vi "gentec-SOLO-PE.Query Configuration.vi"(8 "error in (no error)":errorcluster, 11 "VISA Refnum in":refnum<visa-resource-name>) -> (0 "error out":errorcluster, 1 "Configuration":T1 {"Reference Value" format="%.6f"; "Lower Bond" format="%.6f"; "Upper Bound" format="%.6f"; "Resolution" format="%.7f"; "Max energy (Joulemeter)" format="%.6f"; "Max Power (Joulemeter)" format="%.6f"; "Offset 2" format="%.6f"; "Multiplier 2" format="%.6f"; "Offset 1" format="%.6f"; "Multiplier 1" format="%.6f"; "Zero Offset" format="%.6f"; "Trig Level" format="%.6f"; "Current Scale" items=["Auto", "1 pJ", "3 pJ", "10 pJ", "30 pJ", "100 pJ", "300 pJ", "1 nJ", "3 nJ", "10 nJ", "30 nJ", "100 nJ", "300 nJ", "1 uJ", "3 uJ", "10 uJ", "30 uJ", "100 uJ", "300 uJ", "1 mJ", "3 mJ", "10 mJ", "30 mJ", "100 mJ", "300 mJ", "1 J", "3 J", "10 J", "30 J", "100 J", "300 J", "1 kJ", "3 kJ", "10 kJ", "30 kJ", "100 kJ", "300 kJ", "1 MJ", "3 MJ", "10 MJ", "30 MJ", "100 MJ", "300 MJ"]; "Scale Max Energy" items=["Auto", "1 pJ", "3 pJ", "10 pJ", "30 pJ", "100 pJ", "300 pJ", "1 nJ", "3 nJ", "10 nJ", "30 nJ", "100 nJ", "300 nJ", "1 uJ", "3 uJ", "10 uJ", "30 uJ", "100 uJ", "300 uJ", "1 mJ", "3 mJ", "10 mJ", "30 mJ", "100 mJ", "300 mJ", "1 J", "3 J", "10 J", "30 J", "100 J", "300 J", "1 kJ", "3 kJ", "10 kJ", "30 kJ", "100 kJ", "300 kJ", "1 MJ", "3 MJ", "10 MJ", "30 MJ", "100 MJ", "300 MJ"]; "Scale Min Energy" items=["Auto", "1 pJ", "3 pJ", "10 pJ", "30 pJ", "100 pJ", "300 pJ", "1 nJ", "3 nJ", "10 nJ", "30 nJ", "100 nJ", "300 nJ", "1 uJ", "3 uJ", "10 uJ", "30 uJ", "100 uJ", "300 uJ", "1 mJ", "3 mJ", "10 mJ", "30 mJ", "100 mJ", "300 mJ", "1 J", "3 J", "10 J", "30 J", "100 J", "300 J", "1 kJ", "3 kJ", "10 kJ", "30 kJ", "100 kJ", "300 kJ", "1 MJ", "3 MJ", "10 MJ", "30 MJ", "100 MJ", "300 MJ"]; "Active Sensitivity" format="%.6f"; "Calibration Sensitivity" format="%.6f"}, 2 "Error":string, 3 "VISA Refnum out":refnum<visa-resource-name>, 4 "Timeout":bool)   [LabVIEW 2014, in "gentec-SOLO-PE - Driver.lvlib"]
doc: "Queries the Configuration."
uses:
  gentec-SOLO-PE - Driver.lvlib
  Type Defs/gentec-SOLO-PE.Configuration Values.ctl
  Type Defs/gentec-SOLO-PE.Scale.ctl
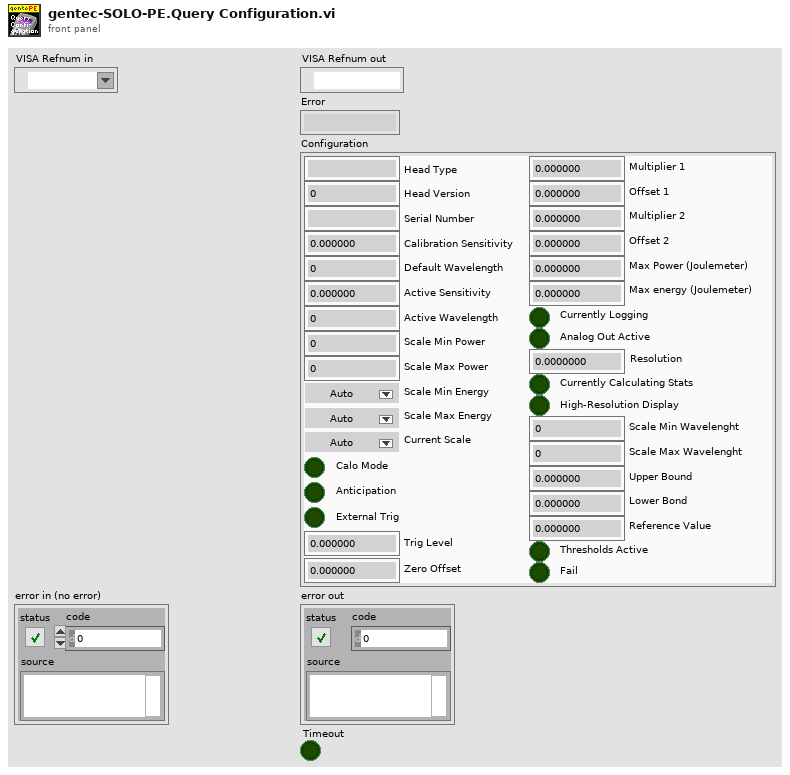
[diagram p1: front panel]
types:
  T1 = typedef "gentec-SOLO-PE - Driver.lvlib/gentec-SOLO-PE.Configuration Values.ctl" = cluster{"Head Type":string, "Head Version":u32, "Serial Number":string, "Calibration Sensitivity":dbl, "Default Wavelength":u32, "Active Sensitivity":dbl, "Active Wavelength":u32, "Scale Min Power":u32, "Scale Max Power":u32, "Scale Min Energy":T2, "Scale Max Energy":T2, "Current Scale":T2, "Calo Mode":bool, "Anticipation":bool, "External Trig":bool, "Trig Level":dbl, "Zero Offset":dbl, "Multiplier 1":dbl, "Offset 1":dbl, "Multiplier 2":dbl, "Offset 2":dbl, "Max Power (Joulemeter)":dbl, "Max energy (Joulemeter)":dbl, "Currently Logging":bool, "Analog Out Active":bool, "Resolution":dbl, "Currently Calculating Stats":bool, "High-Resolution Display":bool, "Scale Min Wavelenght":u32, "Scale Max Wavelenght":u32, "Upper Bound":dbl, "Lower Bond":dbl, "Reference Value":dbl, "Thresholds Active":bool, "Fail":bool}
  T2 = typedef "gentec-SOLO-PE - Driver.lvlib/gentec-SOLO-PE.Scale.ctl" = u32
  T3 = cluster{"Return Parameters[0]":u32, "Return Parameters[1]":u32, "Return Parameters[2]":u32, "Return Parameters[3]":u32, "Return Parameters[4]":u32, "Return Parameters[5]":u32, "Return Parameters[6]":u32, "Return Parameters[7]":u32, "Return Parameters[8]":u32, "Return Parameters[9]":u32, "Return Parameters[10]":u32, "Return Parameters[11]":u32, "Return Parameters[12]":u32, "Return Parameters[13]":u32, "Return Parameters[14]":u32, "Return Parameters[15]":u32, "Return Parameters[16]":u32, "Return Parameters[17]":u32, "Return Parameters[18]":u32, "Return Parameters[19]":u32, "Return Parameters[20]":u32, "Return Parameters[21]":u32, "Return Parameters[22]":u32, "Return Parameters[23]":u32, "Return Parameters[24]":u32, "Return Parameters[25]":u32, "Return Parameters[26]":u32, "Return Parameters[27]":u32, "Return Parameters[28]":u32, "Return Parameters[29]":u32, "Return Parameters[30]":u32, "Return Parameters[31]":u32, "Return Parameters[32]":u32, "Return Parameters[33]":u32, "Return Parameters[34]":u32, "Return Parameters[35]":u32, "Return Parameters[36]":u32, "Return Parameters[37]":u32, "Return Parameters[38]":u32, "Return Parameters[39]":u32, "Return Parameters[40]":u32, "Return Parameters[41]":u32}
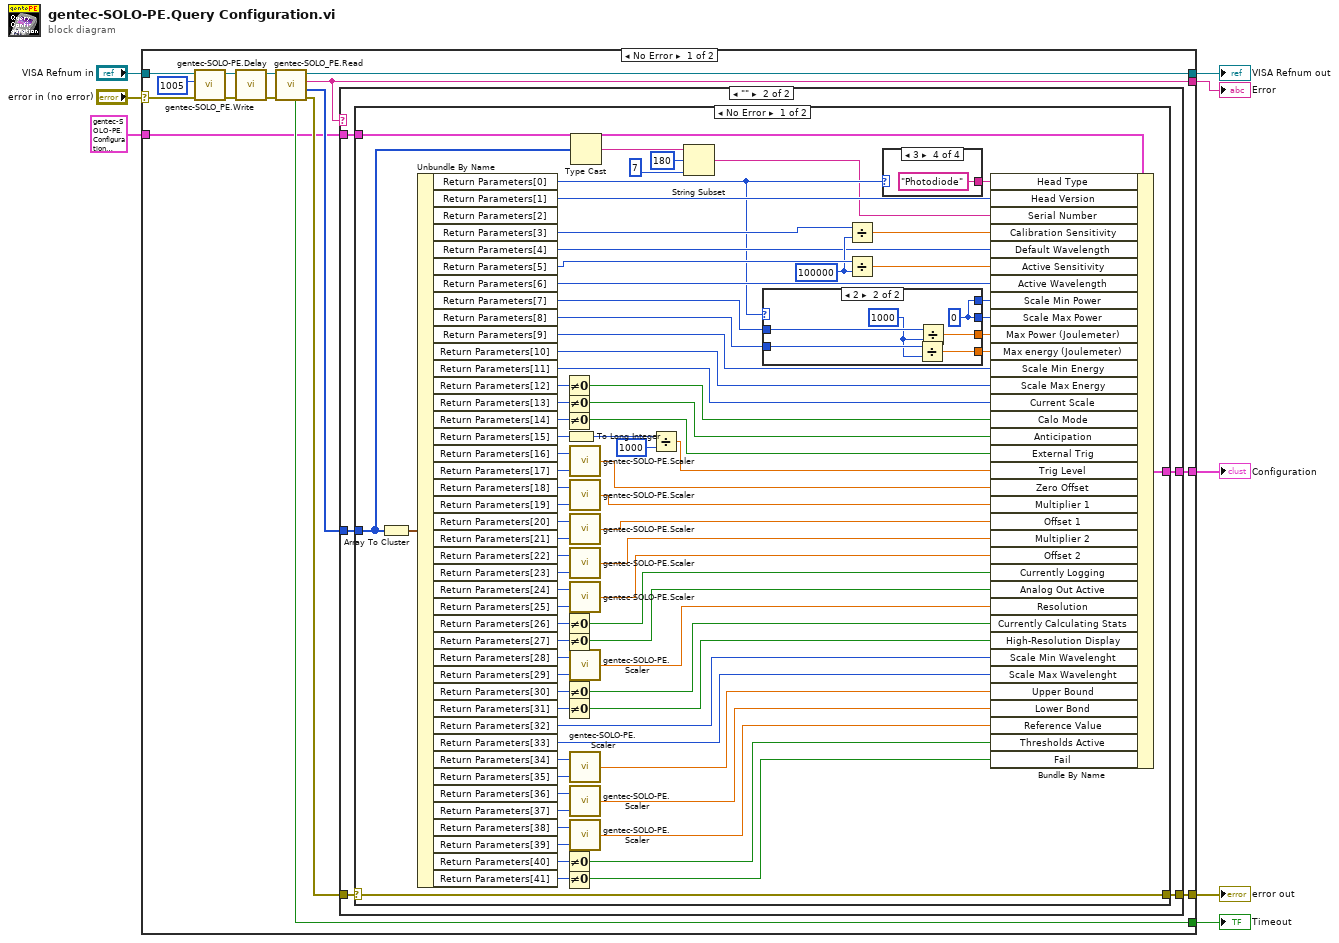
[diagram p0: block diagram]
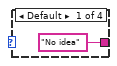
[diagram p3: hidden frame]
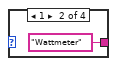
[diagram p4: hidden frame]
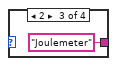
[diagram p5: hidden frame]
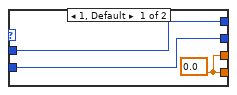
[diagram p6: hidden frame]
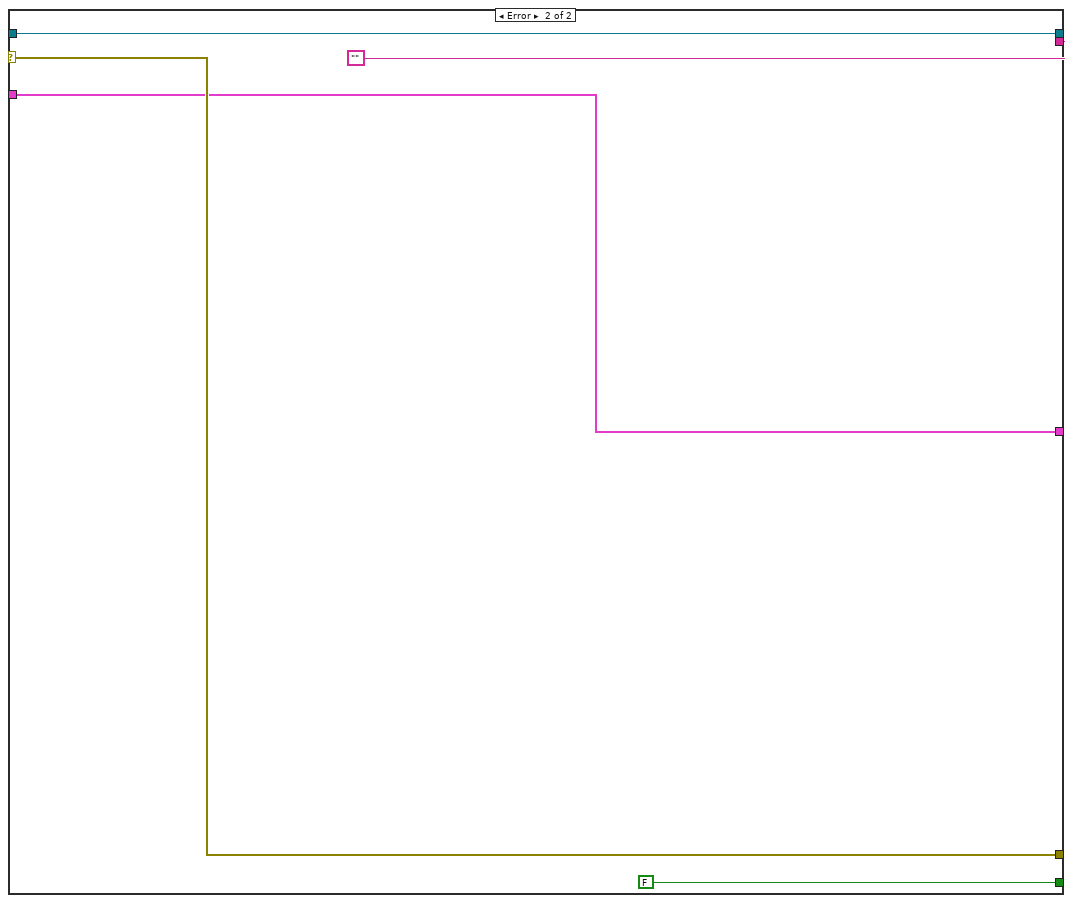
[diagram p8: hidden frame]
diagram:
  n1 = case shown="No Error" "error in (no error)" {
    selector: "error in (no error)" -> [w15 w128]
    tunnel: [w12 w128] -> w8
    tunnel: [w23 w129] -> w7
    tunnel: [w11 ""] -> w6
    tunnel: [w22 FALSE ("Timeout")] -> w5
    tunnel: "VISA Refnum in" -> [w17 w129]
    tunnel: [w10 w125] -> w2
    tunnel: T1 {"Head Type"="", "Head Version"=0, "Serial Number"="", "Calibration Sensitivity"=0.0, "Default Wavelength"=0, "Active Sensitivity"=0.0, "Active Wavelength"=0, "Scale Min Power"=0, "Scale Max Power"=0, "Scale Min Energy"=0, "Scale Max Energy"=0, "Current Scale"=0, "Calo Mode"=FALSE, "Anticipation"=FALSE, "External Trig"=FALSE, "Trig Level"=0.0, "Zero Offset"=0.0, "Multiplier 1"=0.0, "Offset 1"=0.0, "Multiplier 2"=0.0, "Offset 2"=0.0, "Max Power (Joulemeter)"=0.0, "Max energy (Joulemeter)"=0.0, "Currently Logging"=FALSE, "Analog Out Active"=FALSE, "Resolution"=0.0, "Currently Calculating Stats"=FALSE, "High-Resolution Display"=FALSE, "Scale Min Wavelenght"=0, "Scale Max Wavelenght"=0, "Upper Bound"=0.0, "Lower Bond"=0.0, "Reference Value"=0.0, "Thresholds Active"=FALSE, "Fail"=FALSE} ("Configuration") -> [w9 w125]
    frame No Error {
      n2 = call "gentec-SOLO_PE.Write.vi"("error in (no error)"=w15, "Command Handle"=u16 1005, "VISA Refnum in"=w17) -> ("error out"=w20:errorcluster, "VISA Refnum out"=w18:refnum<visa-resource-name>)  [unwired: 7 in]
      n3 = call "gentec-SOLO-PE.Delay.vi"("error in (no error)"=w20, "VISA resource In"=w18) -> ("error out"=w21:errorcluster, "VISA resource Out"=w19:refnum<visa-resource-name>)  [unwired: 4 in]
      n4 = call "gentec-SOLO_PE.Read.vi"("error in (no error)"=w21, "VISA Refnum in"=w19) -> ("error out"=w13:errorcluster, "Return Parameters"=w14:u32[], "Error"=w11:string, "VISA Refnum out"=w23:refnum<visa-resource-name>, "Timeout"=w22:bool)  [unwired: 5 in]
      n5 = case shown="\"\"" w11 {
        tunnel: w14 -> [_ w30]
        tunnel: w13 -> [w25 w29]
        tunnel: [w25 w28] -> w12
        tunnel: w9 -> [w24 w27]
        tunnel: [w24 w26] -> w10
        frame Default {
        }
        frame "" {
          n6 = case shown="No Error" w29 {
            selector: w29 -> [w109 w124]
            tunnel: w30 -> [w34 _]
            tunnel: [w109 w124] -> w28
            tunnel: w27 -> [w44 w123]
            tunnel: [w41 w123] -> w26
            frame No Error {
              w100 = 100000
              n7 = Array To Cluster(array=w34) -> (cluster=w47:T3)
              n8 = Unbundle By Name(w47) -> ("Return Parameters[0]"=w43:u32, "Return Parameters[1]"=w75:u32, "Return Parameters[3]"=w101:u32, "Return Parameters[4]"=w73:u32, "Return Parameters[5]"=w108:u32, "Return Parameters[6]"=w71:u32, "Return Parameters[7]"=w104:u32, "Return Parameters[8]"=w103:u32, "Return Parameters[9]"=w38:u32, "Return Parameters[10]"=w70:u32, "Return Parameters[11]"=w69:u32, "Return Parameters[12]"=w107:u32, "Return Parameters[13]"=w106:u32, "Return Parameters[14]"=w105:u32, "Return Parameters[15]"=w97:u32, "Return Parameters[16]"=w90:u32, "Return Parameters[17]"=w91:u32, "Return Parameters[18]"=w89:u32, "Return Parameters[19]"=w46:u32, "Return Parameters[20]"=w45:u32, "Return Parameters[21]"=w88:u32, "Return Parameters[22]"=w86:u32, "Return Parameters[23]"=w87:u32, "Return Parameters[24]"=w84:u32, "Return Parameters[25]"=w85:u32, "Return Parameters[26]"=w102:u32, "Return Parameters[27]"=w99:u32, "Return Parameters[28]"=w83:u32, "Return Parameters[29]"=w82:u32, "Return Parameters[30]"=w95:u32, "Return Parameters[31]"=w94:u32, "Return Parameters[32]"=w54:u32, "Return Parameters[33]"=w53:u32, "Return Parameters[34]"=w81:u32, "Return Parameters[35]"=w80:u32, "Return Parameters[36]"=w79:u32, "Return Parameters[37]"=w78:u32, "Return Parameters[38]"=w77:u32, "Return Parameters[39]"=w76:u32, "Return Parameters[40]"=w93:u32, "Return Parameters[41]"=w92:u32)  [unwired: 1 out]
              n9 = Not Equal To 0?(x=w107) -> (x != 0?=w68:bool)
              n10 = Not Equal To 0?(x=w106) -> (x != 0?=w67:bool)
              n11 = Not Equal To 0?(x=w105) -> (x != 0?=w66:bool)
              n12 = Not Equal To 0?(x=w102) -> (x != 0?=w59:bool)
              n13 = Not Equal To 0?(x=w99) -> (x != 0?=w58:bool)
              n14 = Not Equal To 0?(x=w95) -> (x != 0?=w56:bool)
              n15 = Not Equal To 0?(x=w94) -> (x != 0?=w55:bool)
              n16 = Not Equal To 0?(x=w93) -> (x != 0?=w49:bool)
              n17 = Not Equal To 0?(x=w92) -> (x != 0?=w48:bool)
              n18 = To Long Integer(number=w97) -> (32bit integer=w98:i32)
              n19 = call "gentec-SOLO-PE.Scaler.vi"("Scaler"=w91, "Value"=w90) -> ("Scaled Value"=w64:dbl)
              n20 = call "gentec-SOLO-PE.Scaler.vi"("Scaler"=w46, "Value"=w89) -> ("Scaled Value"=w63:dbl)
              n21 = call "gentec-SOLO-PE.Scaler.vi"("Scaler"=w88, "Value"=w45) -> ("Scaled Value"=w62:dbl)
              n22 = call "gentec-SOLO-PE.Scaler.vi"("Scaler"=w87, "Value"=w86) -> ("Scaled Value"=w61:dbl)
              n23 = call "gentec-SOLO-PE.Scaler.vi"("Scaler"=w85, "Value"=w84) -> ("Scaled Value"=w60:dbl)
              n24 = call "gentec-SOLO-PE.Scaler.vi"("Scaler"=w82, "Value"=w83) -> ("Scaled Value"=w57:dbl)
              n25 = call "gentec-SOLO-PE.Scaler.vi"("Scaler"=w80, "Value"=w81) -> ("Scaled Value"=w52:dbl)
              n26 = call "gentec-SOLO-PE.Scaler.vi"("Scaler"=w78, "Value"=w79) -> ("Scaled Value"=w51:dbl)
              n27 = call "gentec-SOLO-PE.Scaler.vi"("Scaler"=w76, "Value"=w77) -> ("Scaled Value"=w50:dbl)
              n28 = Type Cast(x=w34) -> (*(type *) &x=w33:string)  [unwired: 1 in]
              n29 = Divide(x=w98, y=1000) -> (x/y=w65:dbl)
              n30 = String Subset(string=w33, offset (0)=180, length (rest)=7 ("length (rest)")) -> (substring=w31:string)
              n31 = case shown="2" w43 {
                tunnel: w104 -> [w116 w121]
                tunnel: w103 -> [w115 w120]
                tunnel: [w116 w122] -> w40
                tunnel: [w115 w122] -> w39
                tunnel: [w114 w119] -> w37
                tunnel: [w114 w118] -> w36
                frame 1, Default {
                  w114 = 0.0
                }
                frame 2 {
                  w117 = 1000
                  w122 = 0
                  n32 = Divide(x=w120, y=w117) -> (x/y=w118:dbl)
                  n33 = Divide(x=w121, y=w117) -> (x/y=w119:dbl)
                }
              }
              n34 = Divide(x=w101, y=w100) -> (x/y=w74:dbl)
              n35 = Divide(x=w108, y=w100) -> (x/y=w72:dbl)
              n36 = case shown="3" w43 {
                tunnel: ["No idea" "Wattmeter" "Joulemeter" "Photodiode"] -> w42
                frame Default {
                }
                frame 1 {
                }
                frame 2 {
                }
                frame 3 {
                }
              }
              n37 = Bundle By Name(cluster=w44, "Head Type"=w42, "Head Version"=w75, "Serial Number"=w31, "Calibration Sensitivity"=w74, "Default Wavelength"=w73, "Active Sensitivity"=w72, "Active Wavelength"=w71, "Scale Min Power"=w40, "Scale Max Power"=w39, "Max Power (Joulemeter)"=w37, "Max energy (Joulemeter)"=w36, "Scale Min Energy"=w38, "Scale Max Energy"=w70, "Current Scale"=w69, "Calo Mode"=w68, "Anticipation"=w67, "External Trig"=w66, "Trig Level"=w65, "Zero Offset"=w64, "Multiplier 1"=w63, "Offset 1"=w62, "Multiplier 2"=w61, "Offset 2"=w60, "Currently Logging"=w59, "Analog Out Active"=w58, "Resolution"=w57, "Currently Calculating Stats"=w56, "High-Resolution Display"=w55, "Scale Min Wavelenght"=w54, "Scale Max Wavelenght"=w53, "Upper Bound"=w52, "Lower Bond"=w51, "Reference Value"=w50, "Thresholds Active"=w49, "Fail"=w48) -> (w41:T1)
            }
            frame Error {
            }
          }
        }
      }
    }
    frame Error {
    }
  }
  "error out" <- w8
  "VISA Refnum out" <- w7
  "Error" <- w6
  "Timeout" <- w5
  "Configuration" <- w2
